vi "Read Sized Payload.vi"(8 "error in (no error)":errorcluster, 9 "timeout ms (100)":i32=100, 11 "TCP in":refnum<k5>) -> (0 "error out":errorcluster, 2 "Payload":string, 3 "TCP":refnum<k5>)   [LabVIEW 2020, in "Vecto.lvlib" / "TCPMessaging.lvclass"]
uses:
  TCPMessaging.lvclass
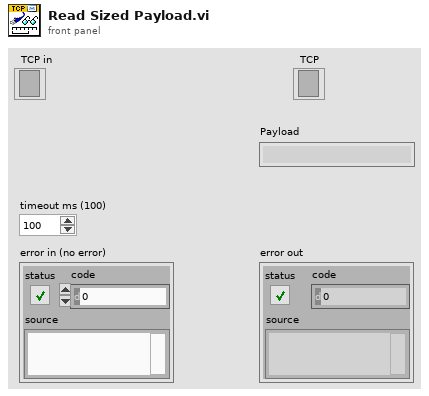
[diagram p1: front panel]
types:
  T1 = enum16{"big-endian, network order", "native, host order", "little-endian"}
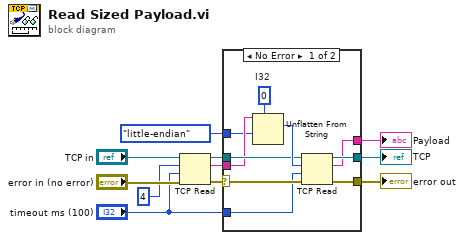
[diagram p0: block diagram]
diagram:
  n1 = TCP Read(connection ID="TCP in", bytes to read=4, error in (no error)="error in (no error)", 9:"timeout ms (100)") -> (connection ID out=w7:refnum<k5>, data out=w3:string, error out=w11:errorcluster)  [unwired: 1 in]
  n2 = case shown="No Error" w11 {
    selector: w11 -> [w21 w22]
    tunnel: w7 -> [w18 w23]
    tunnel: [w17 w23] -> w6
    tunnel: [w16 w22] -> w5
    tunnel: "timeout ms (100)" -> [w15 _]
    tunnel: w3 -> [w14 _]
    tunnel: T1."little-endian" ("byte order (0:big-endian, network order)") -> [w13 _]
    tunnel: [w12 _] -> w1
    frame No Error {
      w20 = 0  # I32
      n3 = Unflatten From String(type=w20, binary string=w14, byte order (0:big-endian, network order)=w13) -> (value=w19:i32)  [unwired: 2 in, 2 out]
      n4 = TCP Read(connection ID=w18, bytes to read=w19, error in (no error)=w21, 9:w15) -> (connection ID out=w17:refnum<k5>, data out=w12:string, error out=w16:errorcluster)  [unwired: 1 in]
    }
    frame Error {
    }
  }
  "TCP" <- w6
  "error out" <- w5
  "Payload" <- w1
